vi "Update.vi"(10 "更新包远端地址":string="/UP/OneStation/V4/一体化微型水质监测站.zip", 11 "测试版？":bool) -> ()   [LabVIEW 2016, in "数据传输系统.lvlib" / "update.lvlib"]
uses:
  update.lvlib
  <vilib>/Utility/miscctls.llb/LVPointTypeDef.ctl
  WebDAV client/WebDAV client.lvclass
panel:
  out "已下载大小":sgl format="%.2f MB"
  out "滑动杆":dbl(slide) scale=0.0..100.0
  in  "取消按钮":bool
  out "last status string":string caption="最近状态字符串"
  out "command":string caption="命令"
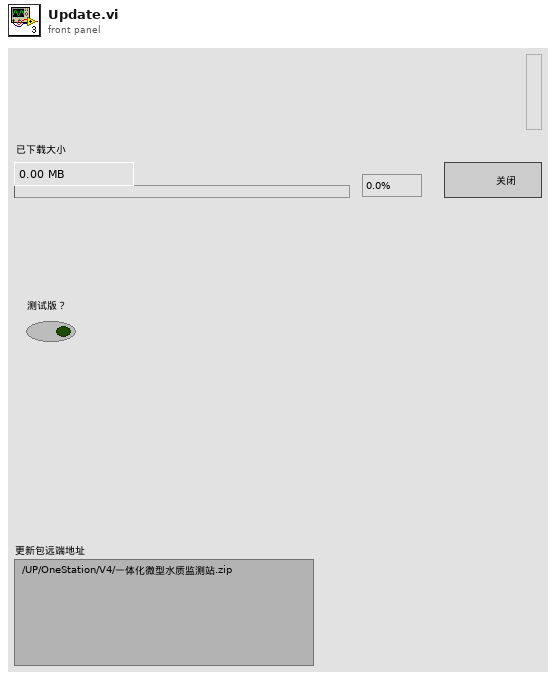
[diagram p1: front panel]
types:
  T1 = typedef "LVPointTypeDef.ctl" = cluster{"Horizontal":i16, "Vertical":i16}
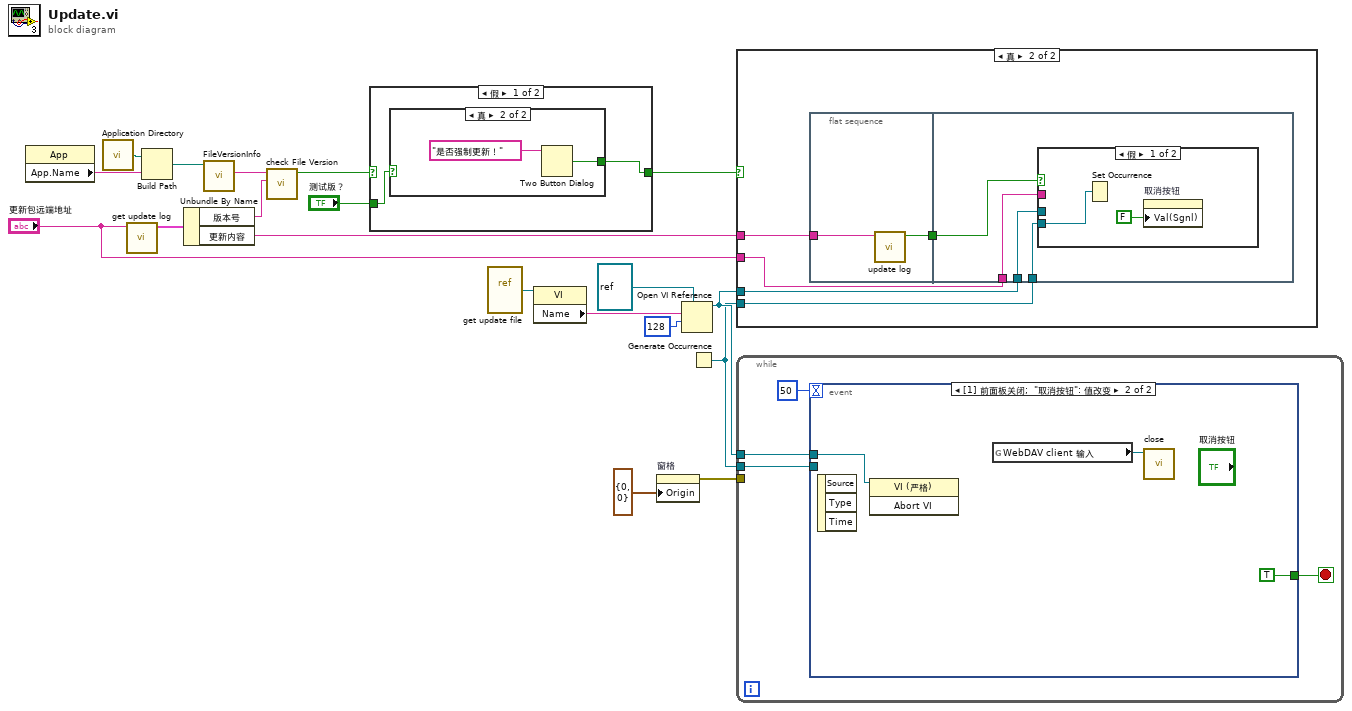
[diagram p0: block diagram]
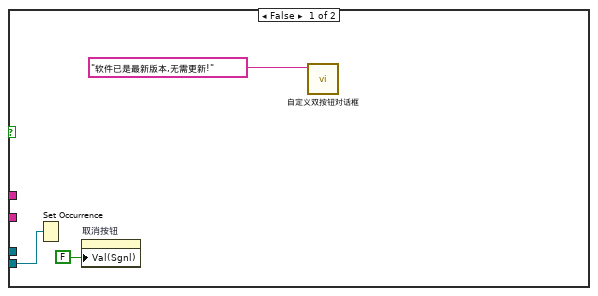
[diagram p4: hidden frame]
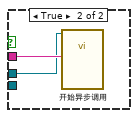
[diagram p5: hidden frame]
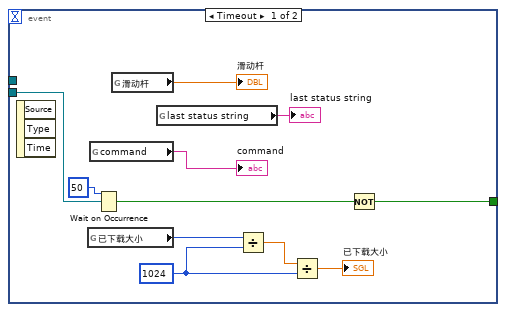
[diagram p6: hidden frame]
diagram:
  n1 = property class="App"() -> ("App.Name"=w19:string)  [unwired: 2 in, 2 out]
  n2 = call <vilib>:"Application Directory.vi"() -> ("Application Directory"=w11:path)
  n3 = call "get update log.vi"("远端地址"="更新包远端地址") -> ("元素"=w12:cluster{"版本号":string, "更新内容":string})  [unwired: 8 in, 2 out]
  n4 = Build Path(base path=w11, name or relative path=w19) -> (appended path=w18:path)
  n5 = Unbundle By Name(w12) -> ("版本号"=w10:string, "更新内容"=w9:string)
  n6 = call <vilib>:"FileVersionInfo.vi"("Application Path in"=w18) -> ("File Version Info"=w17:string)  [unwired: 7 in, 3 out]
  n7 = call "check File Version.vi"("remote File Version Info"=w10, "Local File Version Info"=w17) -> ("new?"=w16:bool)  [unwired: 9 in]
  n8 = case shown="假" w16 {
    selector: w16 -> [_ w24]
    tunnel: [w21 w24] -> w15
    tunnel: "测试版？" -> [w20 _]
    frame False {
      n9 = case shown="真" w20 {
        tunnel: [_ w23] -> w21
        frame False {
        }
        frame True {
          n10 = Two Button Dialog(message="是否强制更新！" ("消息")) -> (T button?=w23:bool)  [unwired: 2 in]
        }
      }
    }
    frame True {
    }
  }
  n11 = vi-ref "get update file.vi"() -> (w5:refnum<vi>)
  n12 = property class="VI"(reference=w5) -> ("Name"=w6:string)  [unwired: 1 in, 2 out]
  n13 = property on="窗格" class="Pane"("Origin"=T1 {"Horizontal"=0, "Vertical"=0} ("原点")) -> (error out=w14:errorcluster)  [unwired: 2 in, 1 out]
  n14 = Open VI Reference(type specifier VI Refnum (for type only)=refnum<vi> refnum, vi path=w6, options=128 ("选项")) -> (vi reference=w4:refnum<vi>)  [unwired: 3 in, 1 out]
  n15 = Generate Occurrence() -> (w3:refnum<k4>)
  n16 = case shown="真" w15 {
    tunnel: w9 -> [_ w32]
    tunnel: "更新包远端地址" -> [_ w30]
    tunnel: w4 -> [_ w29]
    tunnel: w3 -> [w26 w28]
    frame False {
      n17 = Set Occurrence(w26) -> ()
      n18 = property on="取消按钮" class="Bool (严格)"("Val(Sgnl)"=FALSE ("值(信号)")) -> ()  [unwired: 2 in, 2 out]
      n19 = call "自定义双按钮对话框.vi"("消息"="软件已是最新版本,无需更新!") -> ()  [unwired: 10 in, 1 out]
    }
    frame True {
      n20 = flat-sequence {
        tunnel: w32 -> [w34]
        tunnel: [w33] -> w31
        tunnel: w31 -> [w38]
        tunnel: w30 -> [w37]
        tunnel: w29 -> [w36]
        tunnel: w28 -> [w35]
        frame #0 {
          n21 = call "update log.vi"("更新记录"=w34) -> ("check"=w33:bool)  [unwired: 10 in]
        }
        frame #1 {
          n22 = case shown="假" w38 {
            tunnel: w37 -> [_ w42]
            tunnel: w36 -> [_ w41]
            tunnel: w35 -> [w40 _]
            frame False {
              n23 = Set Occurrence(w40) -> ()
              n24 = property on="取消按钮" class="Bool (严格)"("Val(Sgnl)"=FALSE ("值(信号)")) -> ()  [unwired: 2 in, 2 out]
            }
            frame True {
              n25 = call-by-ref "开始异步调用"(reference=w41, "远端地址"=w42) -> ()  [unwired: 11 in, 3 out]
            }
          }
        }
      }
    }
  }
  n26 = while {
    tunnel: w14 -> [_]
    tunnel: w4 -> [w45]
    tunnel: w3 -> [w44]
    stop <- w43 stop-if-true
    n27 = event shown="[1] 前面板关闭;  \"取消按钮\": 值改变" {
      selector: _ -> [_ _]
      dyn-events: _ -> [_ _]
      timeout: 50 -> [_ _]
      tunnel: [w47 TRUE] -> w43
      tunnel: w45 -> [_ w59]
      tunnel: w44 -> [w50 _]
      event Timeout {
        w52 = i64 1024 ("y")
        n28 = event-data() -> ()  [unwired: 1 in, 3 out]
        n29 = global read "更新全局变量.vi" "已下载大小"() -> (w54:i64)
        n30 = global read "更新全局变量.vi" "command"() -> (→"command":string)
        n31 = Wait on Occurrence(2:w50, 3:50 ("毫秒超时(-1)")) -> (0:w48:bool)  [unwired: 1 in]
        n32 = global read "更新全局变量.vi" "滑动杆"() -> (→"滑动杆":dbl)
        n33 = global read "更新全局变量.vi" "last status string"() -> (→"last status string":string)
        n34 = Divide(x=w54, y=w52) -> (x/y=w53:dbl)
        n35 = Divide(x=w53, y=w52) -> (x/y=→"已下载大小":dbl)
        n36 = Not(x=w48) -> (.not. x?=w47:bool)
      }
      event Panel Close; "取消按钮": Value Change {
        n37 = event-data() -> ()  [unwired: 1 in, 3 out]
        n38 = invoke class="VI (严格)" method="Abort VI"(reference=w59) -> ()  [unwired: 2 in, 3 out]
        n39 = global read "更新全局变量.vi" "WebDAV client 输入"() -> (w58:refnum<class "WebDAV client.lvclass">)
        n40 = call-dynamic "close.vi"("WebDAV client 输入"=w58) -> ()  [unwired: 9 in, 2 out]
      }
    }
  }
